vi "Initialize Column Header.vi"(8 "error in (no error)":errorcluster, 11 "Numeric Data Type in":refnum<class "Numeric Data Type.lvclass">) -> (0 "error out":errorcluster, 3 "Numeric Data Type out":refnum<class "Numeric Data Type.lvclass">)   [LabVIEW 2018, in "Numeric Data Type.lvclass"]
uses:
  Numeric Data Type.lvclass
  D:/Code/QControls Extended/DataGrid/DataGrid Configuration/Data Type Classes/Generic/Generic Data Type.lvclass
  Generic/Generic Data Type.lvclass/Generic Data Type.ctl
  Generic/Read Column Header.vi
  Reference Column Header.vi
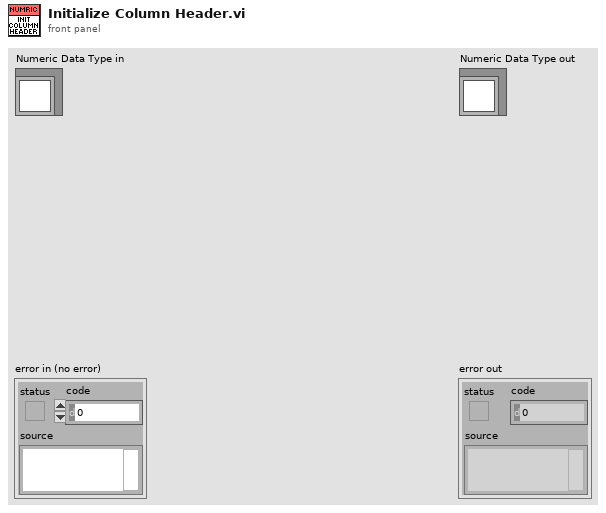
[diagram p1: front panel]
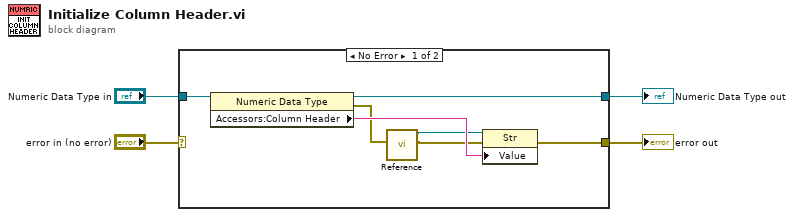
[diagram p0: block diagram]
diagram:
  n1 = case shown="No Error" "error in (no error)" {
    selector: "error in (no error)" -> [_ w13]
    tunnel: [w8 w13] -> w3
    tunnel: [w10 w12] -> w1
    tunnel: "Numeric Data Type in" -> [w11 w12]
    frame No Error {
      n2 = property class="Numeric Data Type"(reference=w11) -> (reference out=w10:refnum<class "Numeric Data Type.lvclass">, error out=w6:errorcluster, "Accessors:Column Header"=w9:string)  [unwired: 1 in]
      n3 = call-poly "Reference.vi"("error in (no error)"=w6) -> ("error out"=w5:errorcluster, "Column Header"=w7:refnum<vi>)  [unwired: 9 in]
      n4 = property class="Str"(reference=w7, error in=w5, "Value"=w9) -> (error out=w8:errorcluster)  [unwired: 1 out]
    }
    frame Error {
    }
  }
  "error out" <- w3
  "Numeric Data Type out" <- w1
